vi "TreePath Destroy.vi"(8 "error in (no error)":errorcluster, 11 "TreePath DVR in":refnum<data-value>) -> (0 "error out":errorcluster)   [LabVIEW 2012, in "MDSplus.lvlib"]
uses:
  <vilib>/MDSplus/Library/MDSplus.lvlib
  <vilib>/MDSplus/Classes/Data_Class/TreeNode_Class/TreePath_Class/TreePath.lvclass
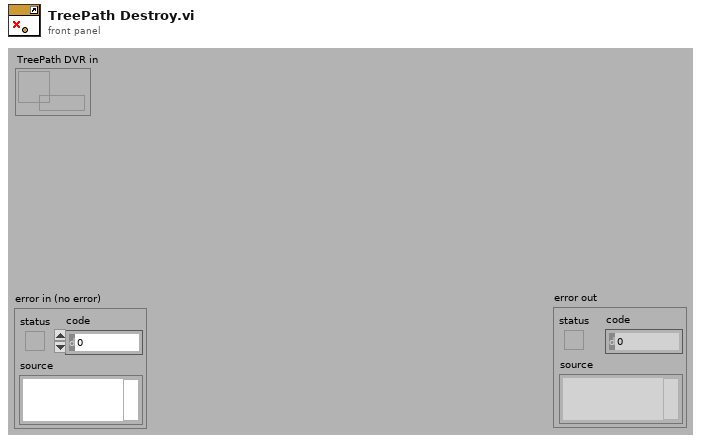
[diagram p1: front panel]
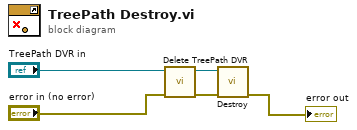
[diagram p0: block diagram]
diagram:
  n1 = call <vilib>:"Delete TreePath DVR.vi"("error in (no error)"="error in (no error)", "TreePath DVR in"="TreePath DVR in") -> ("error out"=w4:errorcluster, "TreePath out"=w5:refnum<class "TreePath.lvclass">)  [unwired: 8 in]
  n2 = call-dynamic "Destroy.vi"("error in (no error)"=w4, "TreePath in"=w5) -> ("error out"=→"error out":errorcluster)  [unwired: 9 in]
